vi "Launch Reader.vi"(8 "error in (no error)":errorcluster, 11 "TCPIP Communications in":refnum<class "TCPIP Communications.lvclass">) -> (0 "error out":errorcluster, 3 "TCPIP Communications out":refnum<class "TCPIP Communications.lvclass">)   [LabVIEW 2015, in "TCPIP Communications Framework.lvlib" / "TCPIP Communications.lvclass"]
uses:
  TCPIP Communications.lvclass
  TCPIP Reader Actor/TCPIP Reader/TCPIP Reader.lvclass
  TCPIP Communications.lvclass/TCPIP Communications.ctl
  <vilib>/ActorFramework/Actor/Actor.lvclass
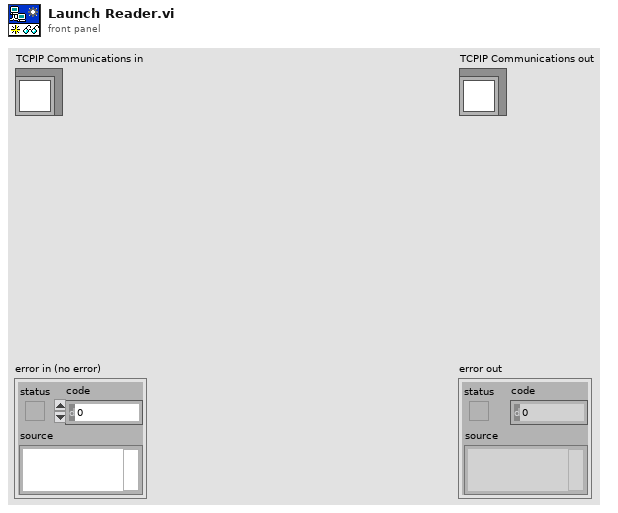
[diagram p1: front panel]
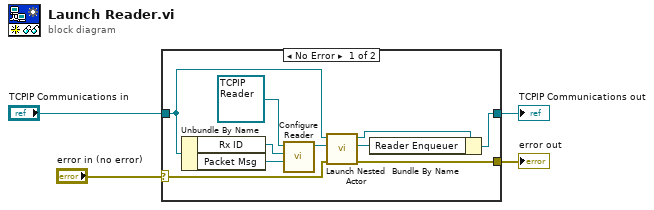
[diagram p0: block diagram]
diagram:
  n1 = case shown="No Error" "error in (no error)" {
    selector: "error in (no error)" -> [w10 w16]
    tunnel: [w5 w16] -> w3
    tunnel: [w7 w15] -> w1
    tunnel: "TCPIP Communications in" -> [w11 w15]
    frame No Error {
      n2 = Unbundle By Name(w11) -> ("Rx ID"=w13:refnum<k5>, "Packet Msg"=w12:refnum<class "Packet Msg.lvclass">)
      n3 = call "Configure Reader.vi"("Packet Msg"=w12, "Rx ID"=w13, "TCPIP Reader in"=refnum<class "TCPIP Reader.lvclass"> refnum ("TCPIP Reader Actor.lvlib:TCPIP Reader.lvclass")) -> ("TCPIP Reader out"=w9:refnum<class "TCPIP Reader.lvclass">)  [unwired: 8 in]
      n4 = call <vilib>:"Launch Nested Actor.vi"("error in (no error)"=w10, "Nested Actor"=w9, "Caller Actor in"=w11) -> ("error out"=w5:errorcluster, "Nested Actor's Enqueuer"=w6:refnum<class "Message Enqueuer.lvclass">, "Caller Actor out"=w8:refnum<class "TCPIP Communications.lvclass">)  [unwired: 6 in]
      n5 = Bundle By Name(cluster=w8, "Reader Enqueuer"=w6) -> (w7:refnum<class "TCPIP Communications.lvclass">)
    }
    frame Error {
    }
  }
  "error out" <- w3
  "TCPIP Communications out" <- w1
